vi "Log Write.vi"(0 "Error In":errorcluster, 1 "Write Header":bool, 5 "Log Handle In":T1, 7 "Trajectory In":refnum<data-value>, 9 "State Estimate In":refnum<data-value>, 11 "Measurement In":refnum<data-value>, 12 "Controller Data In":refnum<data-value>, 13 "Balance In":refnum<data-value>) -> (3 "Logged Events":string[](array[string]), 4 "Error Out":errorcluster, 6 "Log Handle Out":T1, 8 "Trajectory Out":refnum<data-value>, 10 "State Estimate Out":refnum<data-value>, 14 "Controller Data Out":refnum<data-value>, 15 "Measurement Out":refnum<data-value>)   [LabVIEW 2021]
uses:
  State Estimator/Measurements.ctl
  IMU/IMU Data.ctl
  Steering Motor Encoder/Steering Motor Encoder Data.ctl
  GNSS/GNSS Data.ctl
  State Estimator/State Estimate.ctl
  Log Handle.ctl
  Controller Data.ctl
  Drive Motor/Drive Motor Data.ctl
  Steering Motor/Steering Motor Data.ctl
  Trajectory Control/Trajectory_Control.ctl
panel:
  out "velocity":dbl
  out "GNSS Data.Speed (m/s)":dbl
  out "rollReference":dbl
  out "Balance Out":refnum<data-value>
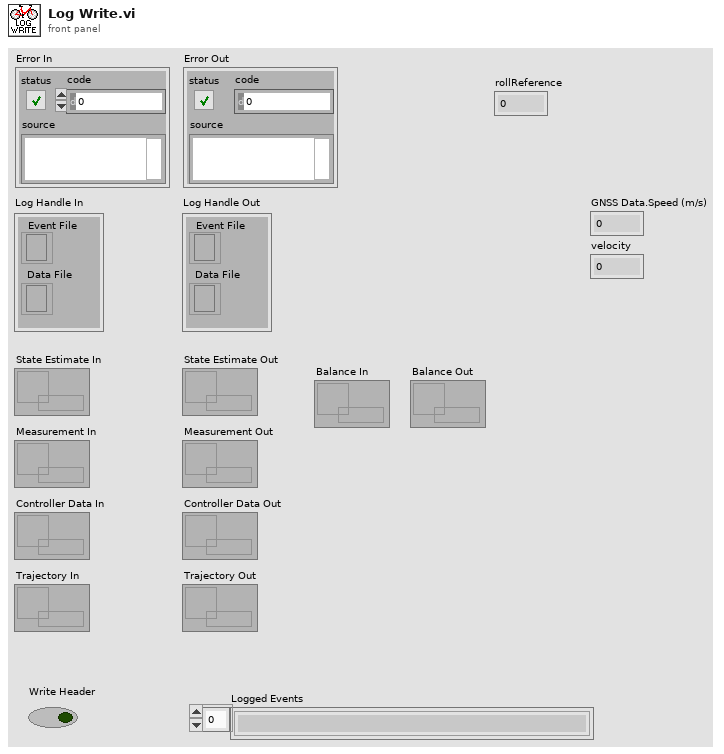
[diagram p1: front panel]
types:
  T1 = typedef "Log Handle.ctl" = cluster{"Data File":refnum<file>, "Event File":refnum<file>}
  T2 = typedef "Trajectory_Control.ctl" = cluster{"Rollref":dbl, "Closestpoint":dbl, "Error1":dbl, "Error2":dbl, "Dpsiref_cont":dbl, "Lateral_cont":dbl, "Heading_cont":dbl, "Reset_traj":dbl, "Iteration":dbl, "E1 limit":u32, "E2 limit":u32}
  T3 = cluster{"Steering Angle Rate":dbl, "rollReference":dbl, "roll":dbl, "rollRate":dbl, "Kp":dbl, "Kd":dbl, "steering_flag":i32}
  T4 = typedef "Measurements.ctl" = cluster{"IMU Data":T5, "Steering Motor Encoder Data":T6, "GNSS Data":T7}
  T5 = typedef "IMU Data.ctl" = cluster{"Gyroscope":cluster{"X (rad/s)":dbl, "Y (rad/s)":dbl, "Z (rad/s)":dbl}, "Accelerometer":cluster{"X (m/s^2)":dbl, "Y (m/s^2)":dbl, "Z (m/s^2)":dbl}, "Flag IMU":dbl}
  T6 = typedef "Steering Motor Encoder Data.ctl" = cluster{"Encoder Position (counts)":i32, "Steering Angle (rad)":dbl, "Flag Steering Encoder":dbl}
  T7 = typedef "GNSS Data.ctl" = cluster{"Latitude (rad)":dbl, "Longitude (rad)":dbl, "Altitude (m)":dbl, "Speed (m/s)":dbl, "Heading (rad)":dbl, "Fix Quality":i32, "Number of Satellites":i32, "Latitude (deg)":dbl, "Longitude (deg)":dbl, "Flag GNSS":dbl}
  T8 = typedef "Controller Data.ctl" = cluster{"Drive Motor Data":T9, "Steering Motor Data":T10}
  T9 = typedef "Drive Motor Data.ctl" = cluster{"Angular Speed (rad/s)":dbl, "Input Current (A)":dbl, "Motor Current (A)":dbl, "MOSFET Temperature (deg C)":dbl, "Reference Speed (rad/s)":dbl, "PI Current (A)":dbl, "Ki":dbl, "Kp":dbl}
  T10 = typedef "Steering Motor Data.ctl" = cluster{"PWM":dbl, "Steering Angle Rate (rad/s)":dbl, "input balancing":dbl}
  T11 = typedef "State Estimate.ctl" = cluster{"X (m)":dbl, "Y (m)":dbl, "Psi (rad)":dbl, "Roll (rad)":dbl, "Roll Rate (rad/s)":dbl, "delta":dbl, "velocity":dbl, "Iterations":dbl}
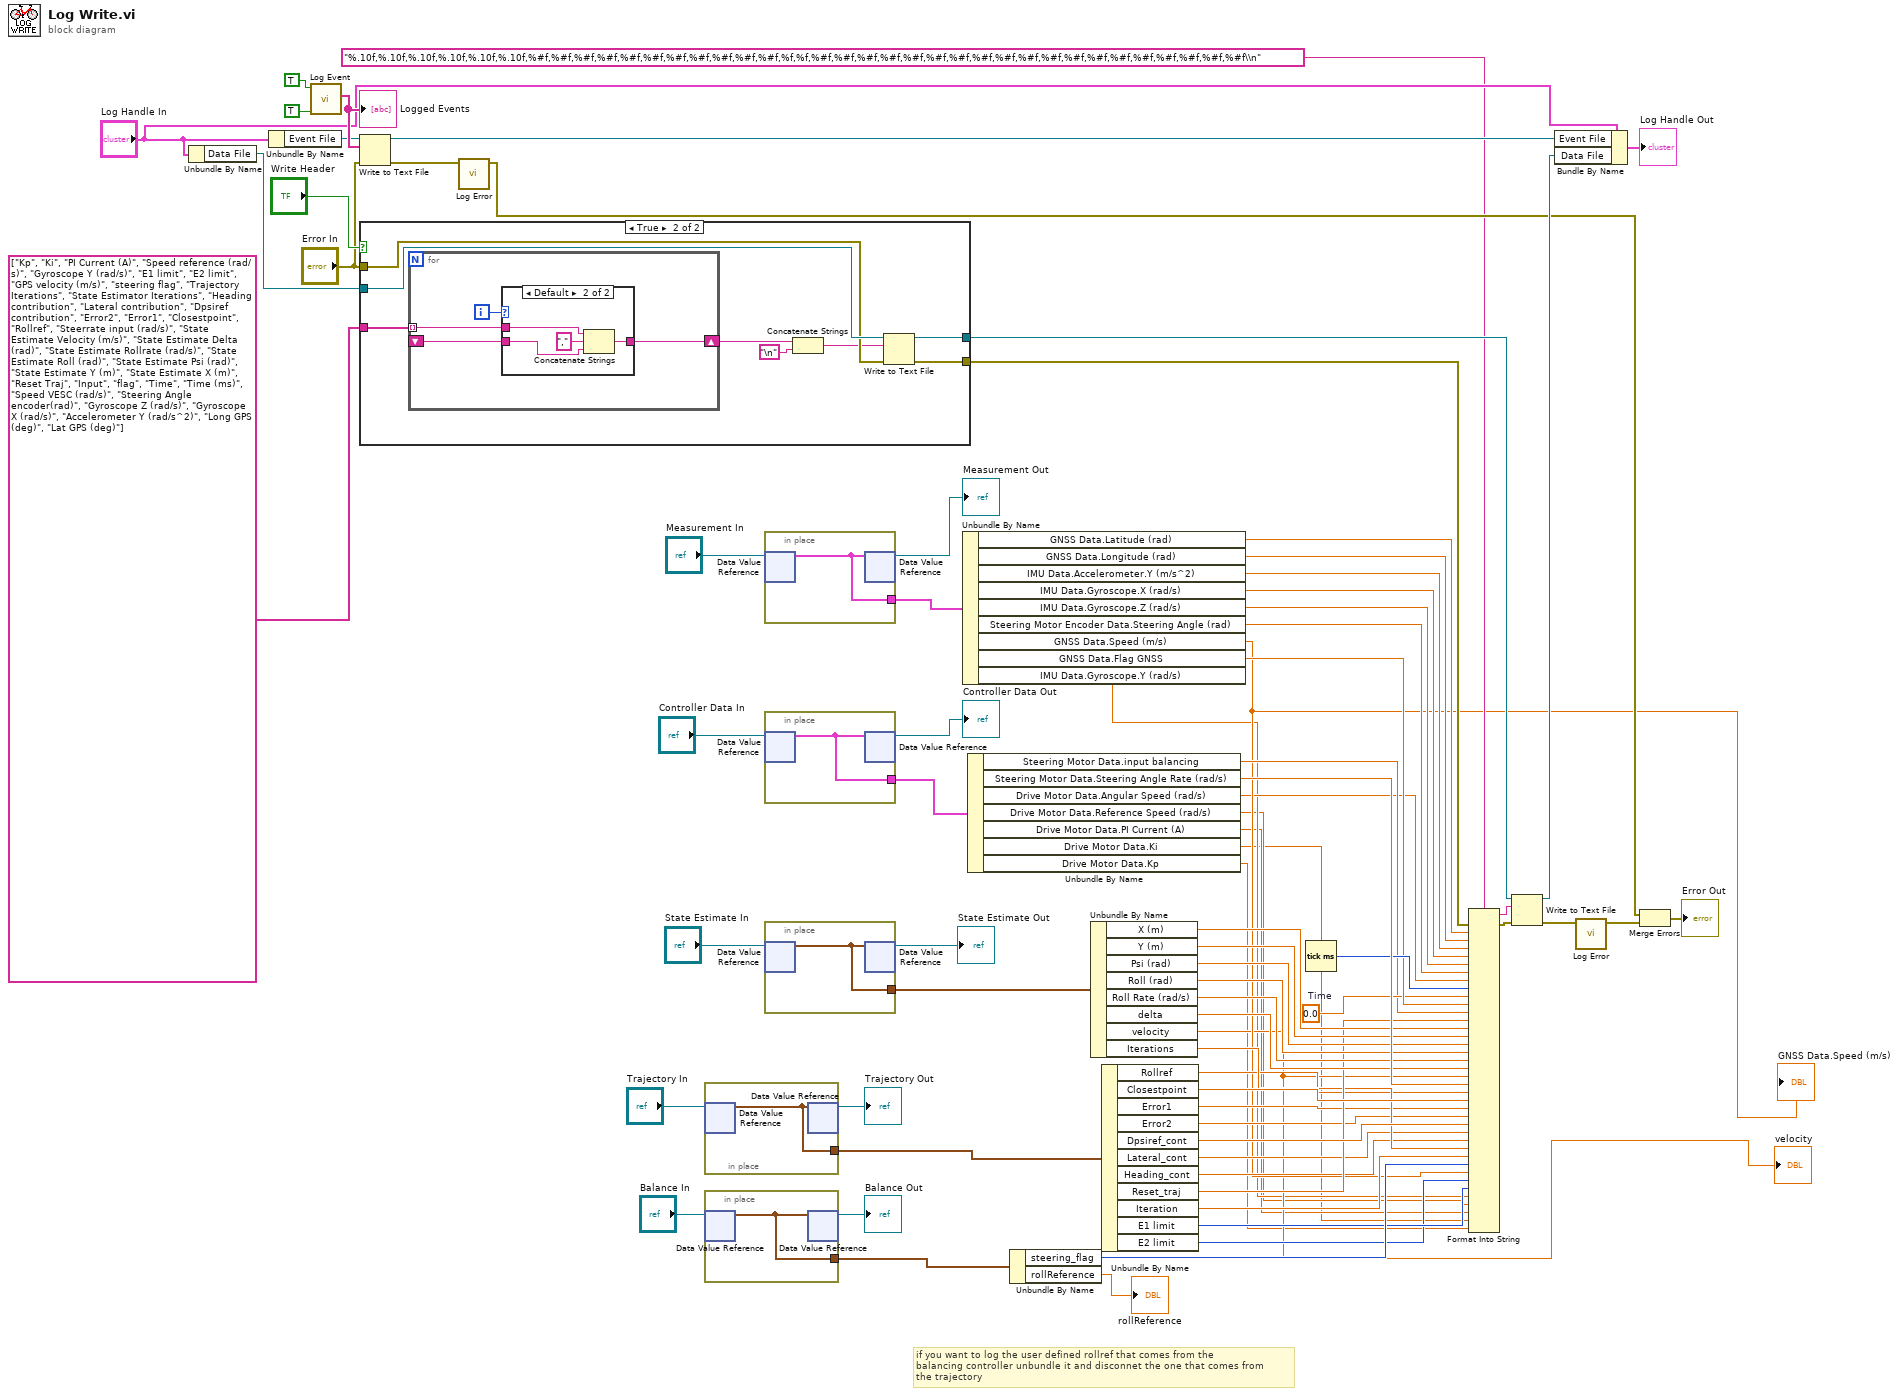
[diagram p0: block diagram]
diagram:
  w25 = 0.0  # Time
  # "if you want to log the user defined rollref that comes from the \nbalancing controller unbundle it and disconnet the one that comes from \nthe trajectory"
  n1 = Unbundle By Name("Log Handle In") -> ("Data File"=w75:refnum<file>)
  n2 = Unbundle By Name("Log Handle In") -> ("Event File"=w67:refnum<file>)
  n3 = call "Log Event.vi"("Clear Log"=TRUE, "Read"=TRUE) -> ("All Events"=w69:string[])  [unwired: 9 in]
  "Logged Events" <- w69
  n4 = Write to Text File(file (use dialog)=w67, text=w69, error in="Error In") -> (refnum out=w64:refnum<file>, error out=w63:errorcluster)  [unwired: 1 in, 1 out]
  n5 = case shown="True" "Write Header" {
    tunnel: string[] ["Kp", "Ki", "PI Current (A)", "Speed reference (rad/s)", "Gyroscope Y (rad/s)", "E1 limit", "E2 limit", "GPS velocity (m/s)", "steering flag", "Trajectory Iterations", "State Estimator Iterations", "Heading contribution", "Lateral contribution", "Dpsiref contribution", "Error2", "Error1", "Closestpoint", "Rollref", "Steerrate input (rad/s)", "State Estimate Velocity (m/s)", "State Estimate Delta (rad)", "State Estimate Rollrate (rad/s)", "State Estimate Roll (rad)", "State Estimate Psi (rad)", "State Estimate Y (m)", "State Estimate X (m)", "Reset Traj", "Input", "flag", "Time", "Time (ms)", "Speed VESC (rad/s)", "Steering Angle encoder(rad)", "Gyroscope Z (rad/s)", "Gyroscope X (rad/s)", "Accelerometer Y (rad/s^2)", "Long GPS (deg)", "Lat GPS (deg)"] ("channel name(s) in (Untitled)") -> [_ w86]
    tunnel: w75 -> [w78 w85]
    tunnel: "Error In" -> [w77 w84]
    tunnel: [w78 w83] -> w73
    tunnel: [w77 w82] -> w72
    frame False {
    }
    frame True {
      n6 = for {
        tunnel: w86 -> [w90] mode=indexing
        shift-right: [w88] -> w81
        shift-left: _ -> [w87]
        i -> [w89]
        n7 = case shown="Default" w89 {
          tunnel: w90 -> [w91 w95]
          tunnel: [w91 w94] -> w88
          tunnel: w87 -> [_ w93]
          frame 0 {
          }
          frame Default {
            n8 = Concatenate Strings(w95, "," ("string"), w93) -> (w94:string)
          }
        }
      }
      n9 = Concatenate Strings(w81, "\n") -> (w80:string)
      n10 = Write to Text File(file (use dialog)=w85, text=w80, error in=w84) -> (refnum out=w83:refnum<file>, error out=w82:errorcluster)  [unwired: 1 in, 1 out]
    }
  }
  n11 = call "Log Error.vi"("Error In"=w63) -> ("Error Out"=w61:errorcluster)  [unwired: 10 in]
  n12 = in-place {
    in-place-border: [w96] -> w29
    n13 = in-place-dvr #1("Trajectory In") -> (w96:T2)  [unwired: 1 out]
    n14 = in-place-dvr #1(w96) -> (→"Trajectory Out":refnum<data-value>)  [unwired: 1 out]
  }
  n15 = in-place {
    in-place-border: [w97] -> w14
    n16 = in-place-dvr #2("Balance In") -> (w97:T3)  [unwired: 1 out]
    n17 = in-place-dvr #2(w97) -> (→"Balance Out":refnum<data-value>)  [unwired: 1 out]
  }
  n18 = in-place {
    in-place-border: [w98] -> w54
    n19 = in-place-dvr #3("Measurement In") -> (w98:T4)  [unwired: 1 out]
    n20 = in-place-dvr #3(w98) -> (→"Measurement Out":refnum<data-value>)  [unwired: 1 out]
  }
  n21 = in-place {
    in-place-border: [w99] -> w41
    n22 = in-place-dvr #4("Controller Data In") -> (w99:T8)  [unwired: 1 out]
    n23 = in-place-dvr #4(w99) -> (→"Controller Data Out":refnum<data-value>)  [unwired: 1 out]
  }
  n24 = in-place {
    in-place-border: [w100] -> w53
    n25 = in-place-dvr #5("State Estimate In") -> (w100:T11)  [unwired: 1 out]
    n26 = in-place-dvr #5(w100) -> (→"State Estimate Out":refnum<data-value>)  [unwired: 1 out]
  }
  n27 = Unbundle By Name(w54) -> ("GNSS Data.Latitude (rad)"=w32:dbl, "GNSS Data.Longitude (rad)"=w52:dbl, "IMU Data.Accelerometer.Y (m/s^2)"=w51:dbl, "IMU Data.Gyroscope.X (rad/s)"=w50:dbl, "IMU Data.Gyroscope.Z (rad/s)"=w49:dbl, "Steering Motor Encoder Data.Steering Angle (rad)"=w48:dbl, "GNSS Data.Speed (m/s)"=w8:dbl, "GNSS Data.Flag GNSS"=w27:dbl, "IMU Data.Gyroscope.Y (rad/s)"=w5:dbl)
  "GNSS Data.Speed (m/s)" <- w8
  n28 = Unbundle By Name(w41) -> ("Steering Motor Data.input balancing"=w23:dbl, "Steering Motor Data.Steering Angle Rate (rad/s)"=w40:dbl, "Drive Motor Data.Angular Speed (rad/s)"=w7:dbl, "Drive Motor Data.Reference Speed (rad/s)"=w4:dbl, "Drive Motor Data.PI Current (A)"=w3:dbl, "Drive Motor Data.Ki"=w2:dbl, "Drive Motor Data.Kp"=w1:dbl)
  n29 = Unbundle By Name(w14) -> ("steering_flag"=w13:i32, "rollReference"=→"rollReference":dbl)
  n30 = Unbundle By Name(w53) -> ("X (m)"=w38:dbl, "Y (m)"=w37:dbl, "Psi (rad)"=w36:dbl, "Roll (rad)"=w35:dbl, "Roll Rate (rad/s)"=w34:dbl, "delta"=w33:dbl, "velocity"=w6:dbl, "Iterations"=w22:dbl)
  "velocity" <- w6
  n31 = Unbundle By Name(w29) -> ("Rollref"=w11:dbl, "Closestpoint"=w28:dbl, "Error1"=w18:dbl, "Error2"=w17:dbl, "Dpsiref_cont"=w26:dbl, "Lateral_cont"=w20:dbl, "Heading_cont"=w19:dbl, "Reset_traj"=w24:dbl, "Iteration"=w21:dbl, "E1 limit"=w10:u32, "E2 limit"=w9:u32)
  n32 = Tick Count (ms)() -> (millisecond timer value=w39:u32)
  n33 = Format Into String(format string="%.10f,%.10f,%.10f,%.10f,%.10f,%.10f,%#f,%#f,%#f,%#f,%#f,%#f,%#f,%#f,%#f,%#f,%#f,%f,%f,%#f,%#f,%#f,%#f,%#f,%#f,%#f,%#f,%#f,%#f,%#f,%#f,%#f,%#f,%#f,%#f,%#f,%#f,%#f\\n", error in=w72, w32, w52, w51, w50, w49, w48, w7, w39, w25, w27, w23, w24, w38, w37, w36, w35, w34, w33, w6, w40, w11, w28, w18, w17, w26, w20, w19, w22, w21, w13, w8, w9, w10, w5, w4, w3, w2, w1) -> (resulting string=w46:string, error out=w45:errorcluster)  [unwired: 1 in]
  n34 = Write to Text File(file (use dialog)=w73, text=w46, error in=w45) -> (refnum out=w65:refnum<file>, error out=w44:errorcluster)  [unwired: 1 in, 1 out]
  n35 = Bundle By Name(cluster="Log Handle In", "Event File"=w64, "Data File"=w65) -> (→"Log Handle Out":T1)
  n36 = call "Log Error.vi"("Error In"=w44) -> ("Error Out"=w62:errorcluster)  [unwired: 10 in]
  n37 = Merge Errors(w61, w62) -> (→"Error Out":errorcluster)
